vi "resetSelection.vi"(8 "error in (no error)":errorcluster, 10 "Selection":i32=-1, 11 "TransactionListUIAdapter in":refnum<class "MultiSelectMCLBAdapter.lvclass">) -> (0 "error out":errorcluster, 3 "TransactionListUIAdapter out":refnum<class "MultiSelectMCLBAdapter.lvclass">)   [LabVIEW 2020, in "MultiSelectMCLBAdapter.lvclass"]
uses:
  MultiSelectMCLBAdapter.lvclass
  MultiSelectMCLBAdapter.lvclass/MultiSelectMCLBAdapter.ctl
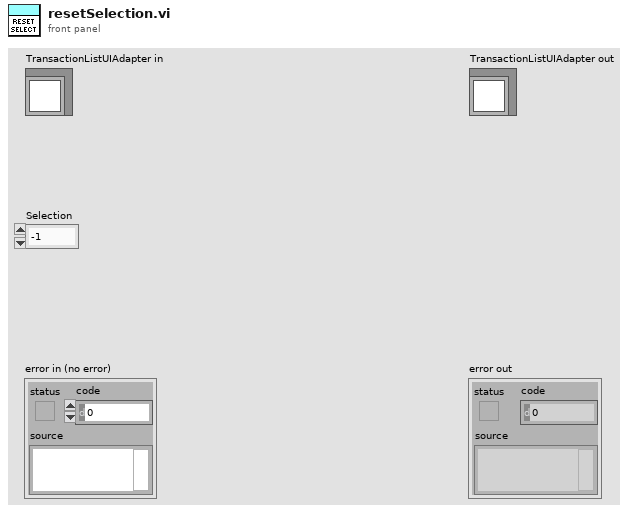
[diagram p1: front panel]
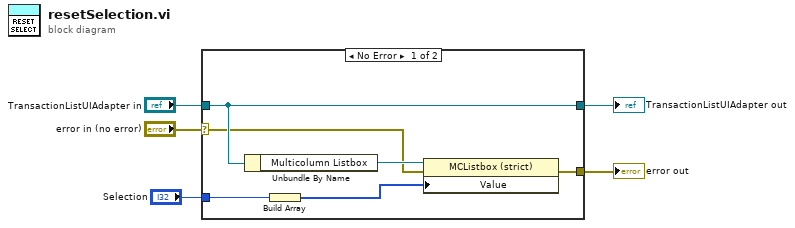
[diagram p0: block diagram]
diagram:
  n1 = case shown="No Error" "error in (no error)" {
    selector: "error in (no error)" -> [w8 w12]
    tunnel: [w9 w13] -> w5
    tunnel: [w11 w12] -> w4
    tunnel: "TransactionListUIAdapter in" -> [w9 w13]
    tunnel: "Selection" -> [w7 _]
    frame No Error {
      n2 = Unbundle By Name(w9) -> ("Multicolumn Listbox"=w10:refnum<vi>)
      n3 = Build Array(w7) -> (w6:i32[])
      n4 = property class="MCListbox (strict)"(reference=w10, error in=w8, "Value"=w6) -> (error out=w11:errorcluster)  [unwired: 1 out]
    }
    frame Error {
    }
  }
  "error out" <- w4
  "TransactionListUIAdapter out" <- w5
